vi "UHR-Fleezers Control (host) - Lorentz v3.vi"() -> ()   [LabVIEW 2014] (continued)
      n59 = call-poly "VISA Configure Serial Port"("VISA resource name"=refnum<visa-resource-name> "COM7", "baud rate (9600)"=u32 115200, "stop bits (10: 1 bit)"=w226) -> ("VISA resource name out"=w225:refnum<visa-resource-name>, "error out"=w224:errorcluster)  [unwired: 4 in, 7 out]
      n60 = call-poly "VISA Configure Serial Port"("VISA resource name"=refnum<visa-resource-name> "COM5", "baud rate (9600)"=u32 115200, "stop bits (10: 1 bit)"=w232) -> ("VISA resource name out"=w229:refnum<visa-resource-name>, "error out"=w228:errorcluster)  [unwired: 4 in, 7 out]
      n61 = call-poly "VISA Configure Serial Port"("VISA resource name"=refnum<visa-resource-name> "COM4", "baud rate (9600)"=u32 115200, "stop bits (10: 1 bit)"=w234) -> ("VISA resource name out"=w231:refnum<visa-resource-name>, "error out"=w230:errorcluster)  [unwired: 4 in, 7 out]
      n62 = call-poly "VISA Configure Serial Port"("VISA resource name"=refnum<visa-resource-name> "COM6", "baud rate (9600)"=u32 115200, "stop bits (10: 1 bit)"=w238) -> ("VISA resource name out"=w236:refnum<visa-resource-name>, "error out"=w237:errorcluster)  [unwired: 4 in, 7 out]
      n63 = call-poly "VISA Configure Serial Port"("VISA resource name"=refnum<visa-resource-name> "COM1") -> ("VISA resource name out"=w220:refnum<visa-resource-name>, "error out"=w240:errorcluster)  [unwired: 5 in, 8 out]
      "Stage Control Serial Error" <- w240
      n64 = local write "Blue Error Out"(w224) -> ()
    }
    frame Enabled {
    }
  }
  n65 = call "IMAQ Create"("Image Name"="APD 1 Image", "Image Type"=w35) -> ("New Image"=w52:T6)  [unwired: 3 in, 1 out]
  n66 = call "IMAQ Create"("Image Name"="APD 2 Image", "Image Type"=w35) -> ("New Image"=w51:T6)  [unwired: 3 in, 1 out]
  n67 = call "IMAQ Create"("Image Name"="APD 3 Image", "Image Type"=w35) -> ("New Image"=w34:T6)  [unwired: 3 in, 1 out]
  n68 = call "IMAQ Create"("Image Name"="Det. X Image", "Image Type"=w35) -> ("New Image"=w50:T6)  [unwired: 3 in, 1 out]
  n69 = call "IMAQ Create"("Image Name"="Det. Y Image", "Image Type"=w35) -> ("New Image"=w49:T6)  [unwired: 3 in, 1 out]
  n70 = Bundle("New Image"=w52, "New Image"=w51, "New Image"=w34, "New Image"=w50, "New Image"=w49) -> (w48:T35)  [unwired: 1 in]
  n71 = xnode "Open FPGA VI Reference"("resource name"=T28 "RIO0") -> ("FPGA VI Reference Out"=w29:T36, "error out"=w28:errorcluster)  [unwired: 1 in]
  n72 = xnode "Invoke Method"("FPGA VI Reference In"=w29, "error in"=w28) -> ("FPGA VI Reference Out"=w9:T36, "error out"=→"FPGA error out":errorcluster)
  n73 = Subtract(x=w7, y="Maximum Delta\n(MHz)") -> (x-y=w5:dbl)
  n74 = Bundle By Name(cluster=T24 {"Minimum"=60.0, "Maximum"=90.0, "Increment"=1.0} ("Min Max Inc"), "Minimum"=w5, "Maximum"=w7) -> (w4:T24)
  n75 = node-c288() -> (w55:T37)  [unwired: 4 in]
  n76 = timed-loop "Run Scripts, including: stage motion" {
    tunnel: w58 -> [w251]
    tunnel: w12 -> [w252]
    tunnel: [w252] -> w57
    tunnel: [w251] -> w56
    timing: w55 -> [_]
    timing-out: [_] -> w54
    tunnel: w46 -> [w250]
    tunnel: w47 -> [w249]
    tunnel: w42 -> [w246]
    tunnel: w41 -> [w245]
    tunnel: w40 -> [w247]
    tunnel: w39 -> [w248]
    tunnel: w31 -> [w244]
    tunnel: w24 -> [w243]
    tunnel: w11 -> [w242]
    tunnel: w10 -> [w241]
    stop <- w253 stop-if-true
    n77 = node-c288() -> ()  [unwired: 1 in, 1 out]
    n78 = event shown="[17] \"Got Bead 1\": Value Change" {
      selector: _ -> [_ _ _ _ _ _ _ _ _ _ _ _ _ _ _ _ _ _ _ _ _ _ _ _ _ _ _ _]
      dyn-events: _ -> [_ _ _ _ _ _ _ _ _ _ _ _ _ _ _ _ _ _ _ _ _ _ _ _ _ _ _ _]
      timeout: _ -> [_ _ _ _ _ _ _ _ _ _ _ _ _ _ _ _ _ _ _ _ _ _ _ _ _ _ _ _]
      tunnel: ["Set Position" "Move to Position" _ _ _ _ _ _ "Read Harvard" _ _ _ _ _ _ _ _ "Got Bead 1" "Force FB Data\nScript" _ "Got Bead 2" _ "Take Stepping Data" _ "Take Detection Laser\nImage" _ _ _] -> _
      tunnel: [_ _ _ _ _ _ _ _ _ _ _ _ _ _ _ _ _ _ _ _ _ _ _ _ _ _ w1180 _] -> w253
      tunnel: w251 -> [w272 w280 w293 w323 _ _ _ _ _ w460 w494 w520 w552 w641 w670 w802 w829 _ w871 _ _ _ _ _ _ _ _ _]
      tunnel: w252 -> [w273 w281 w294 w324 _ _ _ _ _ w461 w495 w521 w553 w642 w671 w803 w830 _ w872 _ _ _ _ _ _ _ _ _]
      tunnel: w250 -> [_ _ _ _ _ _ _ _ w445 _ _ _ _ _ _ _ _ _ _ _ _ _ _ _ _ _ _ _]
      tunnel: w249 -> [_ _ _ _ _ _ _ _ w444 _ _ _ _ _ _ _ _ _ _ _ _ _ _ _ _ _ _ _]
      tunnel: w248 -> [_ _ _ _ _ _ _ _ _ _ _ _ _ _ _ _ _ _ _ _ _ _ _ _ _ _ _ _]
      tunnel: w247 -> [_ _ _ _ _ _ _ _ _ _ _ _ _ _ _ _ _ _ _ _ _ _ _ _ _ _ _ _]
      tunnel: w246 -> [_ _ _ _ _ _ _ _ _ _ _ _ _ _ _ _ _ _ _ _ _ _ _ _ _ _ _ _]
      tunnel: w245 -> [_ _ _ _ _ _ _ _ _ _ _ _ _ _ _ _ _ _ _ _ _ _ _ _ _ _ _ _]
      tunnel: w244 -> [_ _ _ _ w351 w358 w386 w405 _ _ _ _ _ _ _ _ _ _ _ _ _ _ _ _ _ _ w1179 _]
      tunnel: w243 -> [_ _ _ _ _ _ _ _ _ _ _ _ _ _ _ _ _ _ _ _ _ _ _ _ _ w1046 _ _]
      tunnel: w242 -> [_ _ _ _ _ _ _ _ _ _ _ _ _ _ _ _ _ _ _ _ _ _ _ _ _ _ _ w1190]
      tunnel: w241 -> [_ _ _ _ _ _ _ _ _ _ _ _ _ _ _ _ _ _ _ _ _ _ _ _ _ _ _ w1185]
      tunnel: [_ _ _ _ _ _ _ _ _ _ _ _ _ _ _ _ _ _ _ _ _ "Get New Beads" _ _ _ _ _ _] -> _
      event "Set Position", "Set Position 2", "Set Position 3", "Set Position 4", "Set Position 5", "Set Position 1", "Set Position 6": Value Change {
        n79 = event-data() -> ()  [unwired: 1 in, 5 out]
        n80 = Build Array("Set Position 1", "Set Position 2", "Set Position 3", "Set Position 4", "Set Position 5", "Set Position 6") -> (w271:bool[])
        n81 = Boolean Array To Number(Boolean array=w271) -> (number=w270:u32)
        n82 = Logarithm Base 2(1:w270) -> (0:w262:dbl)
        n83 = call "Read Stage Position.vi"("error in"=w272, "VISA resource name in"=w273) -> ("Current Position"=w277:cluster{dbl, dbl, dbl}, "error out"=w276:errorcluster)  [unwired: 2 out]
        n84 = Decrement(x="Position") -> (x-1=w260:dbl)
        n85 = Greater Or Equal?(x=w262, y=0.0) -> (x >= y?=w263:bool)
        n86 = Cluster To Array(cluster=w277) -> (array=w274:dbl[])
        n87 = local write "Stage Control Serial Error"(w276) -> ()
        n88 = Select(t=w262, s=w263, f=w260) -> (s? t:f=w259:dbl)
        n89 = Increment(x=w259) -> (x+1=w258:dbl)
        n90 = Build Array (concatenate)(w258, w274) -> (w257:dbl[])
        n91 = Replace Array Subset(array="Saved Stage Positions", new element=w257, index (row)=w259) -> (w275:dbl[][])  [unwired: 1 in]
        n92 = local write "Saved Stage Positions"(w275) -> ()
      }
      event "Move to Position": Value Change {
        n93 = event-data() -> ()  [unwired: 1 in, 5 out]
        n94 = flat-sequence {
          tunnel: w281 -> [w285]
          tunnel: w280 -> [w284]
          frame #0 {
            n95 = local read "Saved Stage Positions"() -> (w287:dbl[][])
            n96 = local read "Position"() -> (w286:dbl)
            n97 = local write "Stage Moving"(TRUE ("Stage Moving")) -> ()
            n98 = call "move to saved stage position.vi"("error in"=w284, "Stage VISA resource name in"=w285, "Position"=w286, "Saved Stage Positions"=w287) -> ("error out"=w283:errorcluster)  [unwired: 1 out]
            n99 = local write "Stage Control Serial Error"(w283) -> ()
          }
          frame #1 {
            n100 = call <vilib>:"Beep.vi"() -> ()  [unwired: 3 in, 9 out]
            n101 = local write "Stage Moving"(FALSE ("Stage Moving")) -> ()
          }
        }
      }
      event "Move Cap. 1 (DNA Bottom)": Value Change {
        n102 = event-data() -> ()  [unwired: 1 in, 5 out]
        n103 = local write "Move Cap. 1 (DNA Bottom)"(FALSE ("Move Cap. 1 (DNA Right)")) -> ()
        n104 = flat-sequence {
          tunnel: w293 -> [w296]
          tunnel: w294 -> [w297]
          tunnel: [w297] -> w291
          tunnel: [w296] -> w290
          tunnel: w291 -> [w299]
          tunnel: w290 -> [w298]
          frame #0 {
            n105 = property on="Sample Channel\nFlow" class="Bool (strict)"("Val(Sgnl)"="Cap 1 Samp Flow ON") -> ()  [unwired: 2 in, 2 out]
          }
          frame #1 {
            n106 = local read "Saved Stage Positions"() -> (w309:dbl[][])
            n107 = local write "Stage Moving"(TRUE ("Stage Moving")) -> ()
            n108 = Array Subset(array=w309, index (row)=0 ("index"), length (row)=1 ("length"), index (col)=1 ("index"), length (col)=3 ("length")) -> (w306:dbl[][])
            n109 = Reshape Array(w306, 3 ("dimension size")) -> (w304:dbl[])
            n110 = Array To Cluster(array=w304) -> (cluster=w303:cluster{"[0]":dbl, "[1]":dbl, "[2]":dbl})
            n111 = call "Set Stage Position.vi"("Position"=w303, "error in"=w298, "VISA resource name in"=w299) -> ("error out"=w302:errorcluster)  [unwired: 2 out]
            n112 = local write "Stage Control Serial Error"(w302) -> ()
          }
          frame #2 {
            n113 = local write "Stage Moving"(FALSE ("Stage Moving")) -> ()
            n114 = case shown="True" "Cap 1 Flow ON" {
              frame False {
              }
              frame True {
                n115 = property on="Inject Pump 1" class="Bool (strict)"("Val(Sgnl)"=TRUE ("Value (Signaling)")) -> ()  [unwired: 2 in, 2 out]
              }
            }
            n116 = call <vilib>:"Beep.vi"() -> ()  [unwired: 3 in, 9 out]
          }
          frame #3 {
            n117 = property on="Sample Channel\nFlow" class="Bool (strict)"("Val(Sgnl)"=FALSE ("Value (Signaling)")) -> ()  [unwired: 2 in, 2 out]
            n118 = local read "Cap. 2 BD T1?\n(ADig T1, DNA T2)"() -> (w316:bool)
            n119 = case shown="True" w316 {
              tunnel: "Cap 1 T ON" -> [w318 w319]
              frame False {
                n120 = property on="Trap 1 (ON/OFF)" class="Bool (strict)"("Val(Sgnl)"=w318) -> ()  [unwired: 2 in, 2 out]
              }
              frame True {
                n121 = property on="Trap 2 (ON/OFF)" class="Bool (strict)"("Val(Sgnl)"=w319) -> ()  [unwired: 2 in, 2 out]
              }
            }
            n122 = property on="Got Bead 2" class="Bool"("Key Focus"=TRUE) -> ()  [unwired: 2 in, 2 out]
          }
        }
      }
      event "Move Cap. 2 (ADig Top)": Value Change {
        n123 = event-data() -> ()  [unwired: 1 in, 5 out]
        n124 = local write "Move Cap. 2 (ADig Top)"(FALSE ("Move Cap. 2 (ADig Left)")) -> ()
        n125 = flat-sequence {
          tunnel: w323 -> [w326]
          tunnel: w324 -> [w327]
          tunnel: [w327] -> w321
          tunnel: [w326] -> w320
          tunnel: w321 -> [w330]
          tunnel: w320 -> [w329]
          frame #0 {
            n126 = property on="Sample Channel\nFlow" class="Bool (strict)"("Val(Sgnl)"="Cap 2 Samp Flow ON") -> ()  [unwired: 2 in, 2 out]
          }
          frame #1 {
            w328 = FALSE ("Value (Signaling)")
            n127 = local read "Saved Stage Positions"() -> (w340:dbl[][])
            n128 = local write "Stage Moving"(TRUE ("Stage Moving")) -> ()
            n129 = Array Subset(array=w340, index (row)=1 ("index"), length (row)=1 ("length"), index (col)=1 ("index"), length (col)=3 ("length")) -> (w337:dbl[][])
            n130 = Reshape Array(w337, 3 ("dimension size")) -> (w335:dbl[])
            n131 = property on="Trap 1 (ON/OFF)" class="Bool (strict)"("Val(Sgnl)"=w328) -> ()  [unwired: 2 in, 2 out]
            n132 = property on="Trap 1 (ON/OFF)" class="Bool (strict)"("Val(Sgnl)"=w328) -> ()  [unwired: 2 in, 2 out]
            n133 = Array To Cluster(array=w335) -> (cluster=w334:cluster{"[0]":dbl, "[1]":dbl, "[2]":dbl})
            n134 = call "Set Stage Position.vi"("Position"=w334, "error in"=w329, "VISA resource name in"=w330) -> ("error out"=w333:errorcluster)  [unwired: 2 out]
            n135 = local write "Stage Control Serial Error"(w333) -> ()
          }
          frame #2 {
            n136 = local write "Stage Moving"(FALSE ("Stage Moving")) -> ()
            n137 = call <vilib>:"Beep.vi"() -> ()  [unwired: 3 in, 9 out]
            n138 = case shown="True" "Cap 2 Flow ON" {
              frame False {
              }
              frame True {
                n139 = property on="Inject Pump 3" class="Bool (strict)"("Val(Sgnl)"=TRUE ("Value (Signaling)")) -> ()  [unwired: 2 in, 2 out]
              }
            }
          }
          frame #3 {
            n140 = property on="Sample Channel\nFlow" class="Bool (strict)"("Val(Sgnl)"=FALSE ("Value (Signaling)")) -> ()  [unwired: 2 in, 2 out]
            n141 = case shown="False" "Cap. 2 BD T1?\n(ADig T1, DNA T2)" {
              tunnel: "Cap 2 T ON" -> [w349 w350]
              frame False {
                n142 = property on="Trap 2 (ON/OFF)" class="Bool (strict)"("Val(Sgnl)"=w349) -> ()  [unwired: 2 in, 2 out]
              }
              frame True {
                n143 = property on="Trap 1 (ON/OFF)" class="Bool (strict)"("Val(Sgnl)"=w350) -> ()  [unwired: 2 in, 2 out]
              }
            }
            n144 = property on="Got Bead 1" class="Bool"("Key Focus"=TRUE) -> ()  [unwired: 2 in, 2 out]
          }
        }
      }
      event "Send string\nto Blue Laser": Value Change {
        n145 = event-data() -> ()  [unwired: 1 in, 5 out]
        n146 = flat-sequence {
          tunnel: w351 -> [w352]
          frame #0 {
            n147 = call "serial write macro.vi"("String"="command string", "Delay (ms)"="Delay (ms)", "VISA resource name"=w352) -> ("read buffer"=→"read blue buffer":string, "error out"=→"Blue Error Out":errorcluster)  [unwired: 1 out]
            "command string sent" <- "command string"
          }
          frame #1 {
            n148 = local write "Send string\nto Blue Laser"(FALSE ("Send string")) -> ()
          }
        }
      }
      event "Get Blue Laser State": Value Change {
        n149 = event-data() -> ()  [unwired: 1 in, 5 out]
        n150 = local read "Delay (ms)"() -> (w359:i32)
        n151 = flat-sequence {
          tunnel: w359 -> [w367]
          tunnel: w358 -> [w370]
          tunnel: [w368] -> w363
          tunnel: [w367] -> w362
          tunnel: [w377] -> w361
          tunnel: [w374] -> w360
          tunnel: w363 -> [w375]
          tunnel: w362 -> [w374]
          tunnel: w361 -> [w383]
          tunnel: w360 -> [w381]
          frame #0 {
            w365 = "l?"
            n152 = local write "command string sent"(w365) -> ()
            n153 = call "serial write macro.vi"("String"=w365, "Delay (ms)"=w367, "VISA resource name"=w370) -> ("read buffer"=w366:string, "VISA resource name out"=w368:refnum<visa-resource-name>)  [unwired: 1 out]
            n154 = Decimal String To Number(string=w366) -> (number=w369:i32)  [unwired: 2 in, 1 out]
            n155 = Not Equal To 0?(x=w369) -> (x != 0?=→"Laser On":bool)
            n156 = local write "read blue buffer"(w366) -> ()
          }
          frame #1 {
            w372 = "games?" ("String")
            n157 = local write "command string sent"(w372) -> ()
            n158 = call "serial write macro.vi"("String"=w372, "Delay (ms)"=w374, "VISA resource name"=w375) -> ("read buffer"=w373:string, "VISA resource name out"=w377:refnum<visa-resource-name>)  [unwired: 1 out]
            n159 = Decimal String To Number(string=w373) -> (number=w376:i32)  [unwired: 2 in, 1 out]
            n160 = local write "read blue buffer"(w373) -> ()
            n161 = Not Equal To 0?(x=w376) -> (x != 0?=→"Analog Modulation":bool)
          }
          frame #2 {
            w379 = "gdmes?" ("String")
            n162 = local write "command string sent"(w379) -> ()
            n163 = call "serial write macro.vi"("String"=w379, "Delay (ms)"=w381, "VISA resource name"=w383) -> ("read buffer"=w380:string)  [unwired: 2 out]
            n164 = Decimal String To Number(string=w380) -> (number=w382:i32)  [unwired: 2 in, 1 out]
            n165 = Not Equal To 0?(x=w382) -> (x != 0?=→"Digital Modulation":bool)
            n166 = local write "read blue buffer"(w380) -> ()
          }
          frame #3 {
            n167 = local write "Get Blue Laser State"(FALSE) -> ()
          }
        }
      }
      event "Blue Laser Power (mW)\n(Constant Power Mode)", "Blue Laser Modulation\nPower (mW)": Value Change {
        n168 = event-data() -> ()  [unwired: 1 in, 5 out]
        n169 = flat-sequence {
          tunnel: w386 -> [w392]
          tunnel: [w390] -> w385
          tunnel: w385 -> [w399]
          frame #0 {
            n170 = local read "Delay (ms)"() -> (w391:i32)
            n171 = Concatenate Strings("slmp " ("string"), "Blue Laser Modulation\nPower (mW)") -> (w387:string)
            n172 = call "serial write macro.vi"("String"=w387, "Delay (ms)"=w391, "VISA resource name"=w392) -> ("read buffer"=w388:string, "error out"=w389:errorcluster, "VISA resource name out"=w390:refnum<visa-resource-name>)
            n173 = local write "command string sent"(w387) -> ()
            n174 = local write "read blue buffer"(w388) -> ()
            n175 = local write "Blue Error Out"(w389) -> ()
          }
          frame #1 {
            n176 = local read "Delay (ms)"() -> (w398:i32)
            n177 = Concatenate Strings("p " ("string"), "Blue Laser Power (mW)\n(Constant Power Mode)") -> (w395:string)
            n178 = call "serial write macro.vi"("String"=w395, "Delay (ms)"=w398, "VISA resource name"=w399) -> ("read buffer"=w396:string, "error out"=w397:errorcluster)  [unwired: 1 out]
            n179 = local write "command string sent"(w395) -> ()
            n180 = local write "read blue buffer"(w396) -> ()
            n181 = local write "Blue Error Out"(w397) -> ()
          }
        }
      }
      event "Laser interlacing mode", "Blue Laser Modulation Mode", "Blue Laser ON": Value Change {
        n182 = event-data() -> ()  [unwired: 1 in, 5 out]
        n183 = flat-sequence {
          tunnel: w405 -> [w410]
          tunnel: [w409] -> w402
          tunnel: [w415] -> w404
          tunnel: w402 -> [w418]
          tunnel: w404 -> [w430]
          tunnel: [w424] -> w403
          tunnel: w403 -> [w437]
          frame #0 {
            n184 = local read "Blue Laser ON"() -> (w407:bool)
            n185 = local read "Delay (ms)"() -> (w408:i32)
            n186 = case shown="False" w407 {
              tunnel: ["l0" "l1"] -> w406
              frame False {
              }
              frame True {
              }
            }
            n187 = call "serial write macro.vi"("String"=w406, "Delay (ms)"=w408, "VISA resource name"=w410) -> ("error out"=w411:errorcluster, "VISA resource name out"=w409:refnum<visa-resource-name>)  [unwired: 1 out]
            n188 = local write "Blue Error Out"(w411) -> ()
          }
          frame #1 {
            n189 = local read "Laser interlacing mode"() -> (w420:enum32{"Laser ON", "Laser OFF", "Interlace"})
            n190 = case shown="\"Laser ON\"" w420 {
              tunnel: ["cp" "em" "l0"] -> w414
              frame "Laser ON" {
              }
              frame "Interlace" {
              }
              frame "Laser OFF", Default {
              }
            }
            n191 = local read "Delay (ms)"() -> (w419:i32)
            n192 = call "serial write macro.vi"("String"=w414, "Delay (ms)"=w419, "VISA resource name"=w418) -> ("read buffer"=w416:string, "error out"=w417:errorcluster, "VISA resource name out"=w415:refnum<visa-resource-name>)
            n193 = local write "command string sent"(w414) -> ()
            n194 = local write "read blue buffer"(w416) -> ()
            n195 = local write "Blue Error Out"(w417) -> ()
          }
          frame #2 {
            n196 = case shown="\"Analog Modulation\"" "Blue Laser Modulation Mode" {
              tunnel: ["sdmes 0" "sdmes 1" "sdmes 1"] -> w425
              frame "Analog Modulation" {
              }
              frame "Digital + Analog Modulation" {
              }
              frame "Digital Modulation", Default {
              }
            }
            n197 = local read "Delay (ms)"() -> (w428:i32)
            n198 = call "serial write macro.vi"("String"=w425, "Delay (ms)"=w428, "VISA resource name"=w430) -> ("read buffer"=w426:string, "error out"=w427:errorcluster, "VISA resource name out"=w424:refnum<visa-resource-name>)
            n199 = local write "command string sent"(w425) -> ()
            n200 = local write "read blue buffer"(w426) -> ()
            n201 = local write "Blue Error Out"(w427) -> ()
          }
          frame #3 {
            n202 = local read "Blue Laser Modulation Mode"() -> (w439:string)
            n203 = case shown="\"Digital Modulation\", Default" w439 {
              tunnel: ["sames 1" "sames 1" "sames 0"] -> w435
              frame "Analog Modulation" {
              }
              frame "Digital + Analog Modulation" {
              }
              frame "Digital Modulation", Default {
              }
            }
            n204 = local read "Delay (ms)"() -> (w438:i32)
            n205 = local write "command string sent"(w435) -> ()
            n206 = call "serial write macro.vi"("String"=w435, "Delay (ms)"=w438, "VISA resource name"=w437) -> ("read buffer"=w436:string, "error out"=w434:errorcluster)  [unwired: 1 out]
            n207 = local write "read blue buffer"(w436) -> ()
            n208 = local write "Blue Error Out"(w434) -> ()
          }
        }
      }
      event "Read Harvard": Value Change {
        n209 = event-data() -> ()  [unwired: 1 in, 5 out]
        n210 = Concatenate Strings("write buffer", "\r") -> (w447:string)
        n211 = VISA Write(VISA resource name=w445, write buffer=w447, error in (no error)=w444) -> (VISA resource name out=w456:refnum<visa-resource-name>, error out=w455:errorcluster)  [unwired: 1 out]
        n212 = stacked-sequence {
          tunnel: [w459] -> w454
          tunnel: w456 -> [w459]
          tunnel: w455 -> [w458]
          tunnel: [w458] -> w449
          frame #0 {
            n213 = Wait (ms)(milliseconds to wait=50) -> ()  [unwired: 1 out]
          }
        }
        n214 = property class="Instr"(reference=w454, error in=w449) -> (reference out=w453:refnum<visa-resource-name>, error out=w451:errorcluster, "Serial Settings:Number of Bytes at Serial Port"=w452:u32)
        "Serial Settings:Number of Bytes at Serial Port" <- w452
        n215 = VISA Read(VISA resource name=w453, byte count=w452, error in (no error)=w451) -> (read buffer=w450:string)  [unwired: 3 out]
        "read buffer" <- w450
        n216 = Fract/Exp String To Number(string=w450) -> ()  [unwired: 5 out]
      }
      event "+z", "-z": Value Change {
        n217 = event-data() -> ()  [unwired: 1 in, 5 out]
        n218 = flat-sequence {
          tunnel: w460 -> [w482]
          tunnel: w461 -> [w462]
          frame #0 {
            n219 = call "Read Stage Position.vi"("error in"=w482, "VISA resource name in"=w462) -> ("Current Position"=w467:cluster{dbl, dbl, dbl}, "error out"=w480:errorcluster, "VISA resource name out"=w481:refnum<visa-resource-name>)  [unwired: 1 out]
            n220 = local read "Saved Stage Positions"() -> (w491:dbl[][])
            n221 = Divide(x="z nudge increment (um)", y=1000.0) -> (x/y=w479:dbl)
            n222 = Boolean To (0,1)(Boolean="+z") -> (0, 1=w471:i16)
            n223 = Boolean To (0,1)(Boolean="-z") -> (0, 1=w472:i16)
            n224 = Array Subset(array=w491, index (row)=1 ("index"), length (row)=1 ("length"), index (col)=1 ("index"), length (col)=3 ("length")) -> (w488:dbl[][])
            n225 = Multiply(x=w471, y=w479) -> (x*y=w475:dbl)
            n226 = Multiply(x=w472, y=w479) -> (x*y=w473:dbl)
            n227 = Unbundle(w467) -> (w465:dbl, w464:dbl, w468:dbl)
            n228 = Negate(x=w473) -> (-x=w474:dbl)
            n229 = Reshape Array(w488, 3 ("dimension size")) -> (w486:dbl[])
            n230 = Add(x=w475, y=w474) -> (x+y=w476:dbl)
            n231 = Array To Cluster(array=w486) -> ()  [unwired: 1 out]
            n232 = Add(x=w476, y=w468) -> (x+y=w466:dbl)
            n233 = Bundle(cluster=w467, w465, w464, w466) -> (w463:cluster{dbl, dbl, dbl})
            n234 = call "Set Stage Position.vi"("Position"=w463, "error in"=w480, "VISA resource name in"=w481) -> ("error out"=w485:errorcluster)  [unwired: 2 out]
            n235 = local write "Stage Moving"(TRUE ("Stage Moving")) -> ()
            n236 = local write "Stage Control Serial Error"(w485) -> ()
          }
          frame #1 {
            n237 = local write "Stage Moving"(FALSE ("Stage Moving")) -> ()
          }
        }
      }
      event "-y", "+y": Value Change {
        n238 = event-data() -> ()  [unwired: 1 in, 5 out]
        n239 = flat-sequence {
          tunnel: w494 -> [w518]
          tunnel: w495 -> [w501]
          frame #0 {
            n240 = call "Read Stage Position.vi"("error in"=w518, "VISA resource name in"=w501) -> ("Current Position"=w504:cluster{dbl, dbl, dbl}, "error out"=w516:errorcluster, "VISA resource name out"=w517:refnum<visa-resource-name>)  [unwired: 1 out]
            n241 = Divide(x="y nudge increment (um", y=1000.0) -> (x/y=w515:dbl)
            n242 = Boolean To (0,1)(Boolean="+y") -> (0, 1=w507:i16)
            n243 = Boolean To (0,1)(Boolean="-y") -> (0, 1=w508:i16)
            n244 = Multiply(x=w507, y=w515) -> (x*y=w511:dbl)
            n245 = Multiply(x=w508, y=w515) -> (x*y=w509:dbl)
            n246 = Unbundle(w504) -> (w503:dbl, w498:dbl, w500:dbl)
            n247 = Negate(x=w509) -> (-x=w510:dbl)
            n248 = Add(x=w511, y=w510) -> (x+y=w512:dbl)
            n249 = Add(x=w512, y=w498) -> (x+y=w499:dbl)
            n250 = Bundle(cluster=w504, w503, w499, w500) -> (w502:cluster{dbl, dbl, dbl})
            n251 = call "Set Stage Position.vi"("Position"=w502, "error in"=w516, "VISA resource name in"=w517) -> ("error out"=w497:errorcluster)  [unwired: 2 out]
            n252 = local write "Stage Control Serial Error"(w497) -> ()
            n253 = local write "Stage Moving"(TRUE ("Stage Moving")) -> ()
          }
          frame #1 {
            n254 = local write "Stage Moving"(FALSE ("Stage Moving")) -> ()
          }
        }
      }
      event "-x", "+x": Value Change {
        n255 = event-data() -> ()  [unwired: 1 in, 5 out]
        n256 = flat-sequence {
          tunnel: w520 -> [w544]
          tunnel: w521 -> [w528]
          frame #0 {
            n257 = call "Read Stage Position.vi"("error in"=w544, "VISA resource name in"=w528) -> ("Current Position"=w530:cluster{dbl, dbl, dbl}, "error out"=w542:errorcluster, "VISA resource name out"=w543:refnum<visa-resource-name>)  [unwired: 1 out]
            n258 = Divide(x="x nudge increment (um)", y=1000.0) -> (x/y=w541:dbl)
            n259 = Boolean To (0,1)(Boolean="+x") -> (0, 1=w533:i16)
            n260 = Boolean To (0,1)(Boolean="-x") -> (0, 1=w534:i16)
            n261 = Multiply(x=w533, y=w541) -> (x*y=w537:dbl)
            n262 = Multiply(x=w534, y=w541) -> (x*y=w535:dbl)
            n263 = Unbundle(w530) -> (w522:dbl, w524:dbl, w527:dbl)
            n264 = Negate(x=w535) -> (-x=w536:dbl)
            n265 = Add(x=w537, y=w536) -> (x+y=w538:dbl)
            n266 = Add(x=w538, y=w522) -> (x+y=w523:dbl)
            n267 = Bundle(cluster=w530, w523, w524, w527) -> (w529:cluster{dbl, dbl, dbl})
            n268 = call "Set Stage Position.vi"("Position"=w529, "error in"=w542, "VISA resource name in"=w543) -> ("error out"=w525:errorcluster)  [unwired: 2 out]
            n269 = local write "Stage Control Serial Error"(w525) -> ()
            n270 = local write "Stage Moving"(TRUE ("Stage Moving")) -> ()
          }
          frame #1 {
            n271 = local write "Stage Moving"(FALSE ("Stage Moving")) -> ()
          }
        }
      }
      event "Cal/Data Acq. Spot": Value Change {
        # "Disabled by Ronen - we have our own way of controlling the location of calibration."
        n272 = event-data() -> ()  [unwired: 1 in, 5 out]
        n273 = flat-sequence {
          tunnel: w552 -> [w556]
          tunnel: w553 -> [w557]
          tunnel: [w557] -> w549
          tunnel: [w556] -> w548
          tunnel: w549 -> [w560]
          tunnel: w548 -> [w559]
          tunnel: ["Cal @ (MHz)"] -> w546
          tunnel: [w568] -> w550
          tunnel: w546 -> [w568]
          tunnel: w550 -> [w580]
          tunnel: ["W/ Offset 1"] -> w547
          tunnel: w550 -> [w601]
          tunnel: w547 -> [w599]
          frame #0 {
            n274 = property on="Sample Channel\nFlow" class="Bool (strict)"("Val(Sgnl)"="Daq spot flow on") -> ()  [unwired: 2 in, 2 out]
            n275 = Wait (ms)(milliseconds to wait=u32 250) -> ()  [unwired: 1 out]
          }
          frame #1 {
            n276 = disable-structure shown="Disabled" {
              disable-tunnel: w560 -> [w565 _]
              disable-tunnel: w559 -> [w564 _]
              frame Disabled {
                n277 = local read "Saved Stage Positions"() -> (w562:dbl[][])
                n278 = call "move to saved stage position.vi"("error in"=w564, "Stage VISA resource name in"=w565, "Position"="Cal Stage Position", "Saved Stage Positions"=w562) -> ("error out"=w563:errorcluster)  [unwired: 1 out]
                n279 = local write "Stage Control Serial Error"(w563) -> ()
              }
              frame Enabled {
              }
            }
            n280 = property on="Trap Delta (MHz)" class="DigNum (strict)"("Val(Sgnl)"="Cal @ (MHz)") -> ()  [unwired: 2 in, 2 out]
            n281 = local write "Stage Moving"(TRUE ("Stage Moving")) -> ()
          }
          frame #2 {
            n282 = local write "Stage Moving"(FALSE ("Stage Moving")) -> ()
            n283 = property on="Sample Channel\nFlow" class="Bool (strict)"("Val(Sgnl)"="Flow ON during cal?") -> ()  [unwired: 2 in, 2 out]
            n284 = call <vilib>:"Beep.vi"() -> ()  [unwired: 3 in, 9 out]
          }
          frame #3 {
            n285 = Wait (ms)(milliseconds to wait=u32 1000) -> ()  [unwired: 1 out]
          }
          frame #4 {
            n286 = case shown="True" "Active cal after cal?" {
              frame False {
              }
              frame True {
                n287 = local write "Active Cal"(TRUE ("Active Cal")) -> ()
                n288 = Wait (ms)(milliseconds to wait=u32 8000) -> ()  [unwired: 1 out]
              }
            }
          }
          frame #5 {
            n289 = property on="Save Calibration" class="Bool (strict)"("Val(Sgnl)"=TRUE ("Value (Signaling)")) -> ()  [unwired: 2 in, 2 out]
          }
          frame #6 {
            n290 = Wait (ms)(milliseconds to wait=u32 2000) -> ()  [unwired: 1 out]
          }
          frame #7 {
            # "Check to see if \nsaving done"
            n291 = while {
              stop <- w576 stop-if-true
              n292 = local read "Saving..."() -> (w577:bool)
              n293 = Wait (ms)(milliseconds to wait=u32 100) -> ()  [unwired: 1 out]
              n294 = Not(x=w577) -> (.not. x?=w576:bool)
            }
          }
          frame #8 {
            n295 = case shown="True" "W/ Offset 1" {
              tunnel: w580 -> [_ w581]
              frame False {
              }
              frame True {
                n296 = stacked-sequence {
                  tunnel: w581 -> [_ _ _ _ _ _ _ w598]
                  frame #0 {
                    n297 = property on="Trap Delta (MHz)" class="DigNum (strict)"("Val(Sgnl)"="Offset 1 Start (MHz)") -> ()  [unwired: 2 in, 2 out]
                    n298 = Replace Array Subset(array=u32[] [0] ("Index Values"), new element="Offset 1 Set", index=0) -> (w583:u32[])
                    n299 = property on="Saved AOD Raster Scan Parameter Sets" class="Arr (strict)"("Index Values"=w583) -> ()  [unwired: 2 in, 2 out]
                    n300 = property on="manual raster set" class="Ring (strict)"("Value"="Offset 1 Set") -> ()  [unwired: 2 in, 2 out]
                  }
                  frame #1 {
                    n301 = Wait (ms)(milliseconds to wait=u32 200) -> ()  [unwired: 1 out]
                  }
                  frame #2 {
                    n302 = property on="Load parameters" class="Bool (strict)"("Val(Sgnl)"=TRUE ("Value (Signaling)")) -> ()  [unwired: 2 in, 2 out]
                  }
                  frame #3 {
                    n303 = Wait (ms)(milliseconds to wait=u32 200) -> ()  [unwired: 1 out]
                  }
                  frame #4 {
                    n304 = property on="Trap Raster Scan" class="Bool (strict)"("Val(Sgnl)"=TRUE ("Value (Signaling)")) -> ()  [unwired: 2 in, 2 out]
                  }
                  frame #5 {
                    n305 = Wait (ms)(milliseconds to wait=u32 2000) -> ()  [unwired: 1 out]
                  }
                  frame #6 {
                    n306 = while {
                      stop <- w595 stop-if-true
                      n307 = local read "Raster Scanning..."() -> (w597:bool)
                      n308 = local read "Saving..."() -> (w593:bool)
                      n309 = Wait (ms)(milliseconds to wait=u32 100) -> ()  [unwired: 1 out]
                      n310 = Not(x=w593) -> (.not. x?=w592:bool)
                      n311 = Not(x=w597) -> (.not. x?=w594:bool)
                      n312 = And(x=w594, y=w592) -> (x .and. y?=w595:bool)
                    }
                  }
                  frame #7 {
                    n313 = property on="Trap Delta (MHz)" class="DigNum (strict)"("Val(Sgnl)"=w598) -> ()  [unwired: 2 in, 2 out]
                  }
                }
              }
            }
          }
          frame #9 {
            n314 = local read "Save ave N"() -> (w600:dbl)
            n315 = case shown="True" "W/ Offset 2" {
              tunnel: w601 -> [_ w608]
              tunnel: w600 -> [_ w607]
              tunnel: w599 -> [w603 _]
              frame False {
                n316 = case shown="False" w603 {
                  frame False {
                    n317 = Multiply(x="Cal read wait (s)", y=u32 1000 ("milliseconds to wait")) -> (x*y=w605:u32)
                    n318 = Wait (ms)(milliseconds to wait=w605) -> ()  [unwired: 1 out]
                  }
                  frame True {
                  }
                }
              }
              frame True {
                n319 = stacked-sequence {
                  tunnel: w608 -> [_ _ _ _ _ _ _ _ _ w629 _ _]
                  tunnel: w607 -> [_ _ _ _ _ _ _ _ _ w627 _ _]
                  frame #0 {
                    n320 = property on="Save ave N" class="DigNum (strict)"("Val(Sgnl)"=1.0 ("Value (Signaling)")) -> ()  [unwired: 2 in, 2 out]
                  }
                  frame #1 {
                    n321 = Wait (ms)(milliseconds to wait=u32 500) -> ()  [unwired: 1 out]
                  }
                  frame #2 {
                    n322 = property on="Trap Delta (MHz)" class="DigNum (strict)"("Val(Sgnl)"="Offset 2 Start (MHz)") -> ()  [unwired: 2 in, 2 out]
                    n323 = Replace Array Subset(array=u32[] [0] ("Index Values"), new element="Offset 2 Set", index=0) -> (w613:u32[])
                    n324 = property on="Saved AOD Raster Scan Parameter Sets" class="Arr (strict)"("Index Values"=w613) -> ()  [unwired: 2 in, 2 out]
                  }
                  frame #3 {
                    n325 = Wait (ms)(milliseconds to wait=u32 500) -> ()  [unwired: 1 out]
                  }
                  frame #4 {
                    n326 = property on="Load parameters" class="Bool (strict)"("Val(Sgnl)"=TRUE ("Value (Signaling)")) -> ()  [unwired: 2 in, 2 out]
                  }
                  frame #5 {
                    n327 = Wait (ms)(milliseconds to wait=u32 500) -> ()  [unwired: 1 out]
                  }
                  frame #6 {
                    n328 = property on="Trap Raster Scan" class="Bool (strict)"("Val(Sgnl)"=TRUE ("Value (Signaling)")) -> ()  [unwired: 2 in, 2 out]
                  }
                  frame #7 {
                    n329 = Wait (ms)(milliseconds to wait=u32 2000) -> ()  [unwired: 1 out]
                  }
                  frame #8 {
                    n330 = while {
                      stop <- w622 stop-if-true
                      n331 = local read "Raster Scanning..."() -> (w625:bool)
                      n332 = local read "Saving..."() -> (w623:bool)
                      n333 = Wait (ms)(milliseconds to wait=u32 100) -> ()  [unwired: 1 out]
                      n334 = Not(x=w623) -> (.not. x?=w621:bool)
                      n335 = Not(x=w625) -> (.not. x?=w624:bool)
                      n336 = And(x=w624, y=w621) -> (x .and. y?=w622:bool)
                    }
                  }
                  frame #9 {
                    n337 = property on="Trap Delta (MHz)" class="DigNum (strict)"("Val(Sgnl)"=w629) -> ()  [unwired: 2 in, 2 out]
                    n338 = property on="Saved AOD Raster Scan Parameter Sets" class="Arr (strict)"("Index Values"=u32[] [0]) -> ()  [unwired: 2 in, 2 out]
                    n339 = property on="Save ave N" class="DigNum (strict)"("Val(Sgnl)"=w627) -> ()  [unwired: 2 in, 2 out]
                  }
                  frame #10 {
                    n340 = Wait (ms)(milliseconds to wait=u32 500) -> ()  [unwired: 1 out]
                  }
                  frame #11 {
                    n341 = property on="Load parameters" class="Bool (strict)"("Val(Sgnl)"=TRUE ("Value (Signaling)")) -> ()  [unwired: 2 in, 2 out]
                  }
                }
              }
            }
          }
          frame #10 {
            # "Added by Ronen for flow calibration"
            n342 = case shown="True" "Flow based calibration?" {
              frame False {
              }
              frame True {
                n343 = stacked-sequence {
                  frame #0 {
                    n344 = local write "Flow Cal"(TRUE) -> ()
                  }
                  frame #1 {
                  }
                  frame #2 {
                    n345 = Wait (ms)(milliseconds to wait=u32 8000) -> ()  [unwired: 1 out]
                  }
                }
              }
            }
          }
          frame #11 {
            n346 = property on="Read Cal" class="Bool (strict)"("Val(Sgnl)"=TRUE ("Value (Signaling)")) -> ()  [unwired: 2 in, 2 out]
          }
          frame #12 {
            n347 = Wait (ms)(milliseconds to wait=u32 1000) -> ()  [unwired: 1 out]
          }
          frame #13 {
            n348 = property on="Fish for Tether" class="Bool (strict)"("Val(Sgnl)"="Fish after cal?") -> ()  [unwired: 2 in, 2 out]
          }
        }
        n349 = local write "Cal/Data Acq. Spot"(FALSE ("Cal/Data Acq. Spot")) -> ()
      }
      event "Dump Beads": Value Change {
        n350 = event-data() -> ()  [unwired: 1 in, 5 out]
        n351 = flat-sequence {
          tunnel: ["Dump spot flow on?"] -> w638
          tunnel: [w649] -> w639
          tunnel: w638 -> [w649]
          tunnel: w642 -> [w654]
          tunnel: w641 -> [w653]
          tunnel: [w651] -> w640
          tunnel: w639 -> [w651]
          tunnel: w640 -> [w664]
          frame #0 {
            w643 = FALSE ("Value (Signaling)")
            n352 = local read "Saving..."() -> (w645:bool)
            n353 = local write "Dump Beads"(FALSE ("Dump Beads")) -> ()
            n354 = property on="Inject Pump 3" class="Bool (strict)"("Val(Sgnl)"=w643) -> ()  [unwired: 2 in, 2 out]
            n355 = property on="Inject Pump 1" class="Bool (strict)"("Val(Sgnl)"=w643) -> ()  [unwired: 2 in, 2 out]
            n356 = local write "Stop Saving"(w645) -> ()
          }
          frame #1 {
            w646 = FALSE ("Fl. Triggered...")
            n357 = case shown="True" "Dump spot flow on?" {
              frame False {
              }
              frame True {
                n358 = property on="Sample Channel\nFlow" class="Bool (strict)"("Val(Sgnl)"=TRUE ("Stage Moving")) -> ()  [unwired: 2 in, 2 out]
              }
            }
            n359 = local write "Fl. Triggered..."(w646) -> ()
            n360 = local write "Tether"(w646) -> ()
            n361 = property on="Green Laser ON" class="Bool (strict)"("Val(Sgnl)"=w646) -> ()  [unwired: 2 in, 2 out]
            n362 = property on="Trap Pos. FB ON" class="Bool (strict)"("Val(Sgnl)"=w646) -> ()  [unwired: 2 in, 2 out]
            n363 = property on="Trap Trig. Fl." class="Bool (strict)"("Val(Sgnl)"=w646) -> ()  [unwired: 2 in, 2 out]
            n364 = property on="Fl. Triggered..." class="Bool (strict)"("Val(Sgnl)"=w646) -> ()  [unwired: 2 in, 2 out]
            n365 = property on="Dip for Protein" class="Bool (strict)"("Val(Sgnl)"=w646) -> ()  [unwired: 2 in, 2 out]
            n366 = property on="Pause dwell" class="Bool (strict)"("Val(Sgnl)"=w646) -> ()  [unwired: 2 in, 2 out]
          }
          frame #2 {
            n367 = property on="Trap Pos. FB Offset Factor" class="DigNum (strict)"("Val(Sgnl)"=i64 0 ("Value (Signaling)")) -> ()  [unwired: 2 in, 2 out]
          }
          frame #3 {
            n368 = local read "Saved Stage Positions"() -> (w655:dbl[][])
            n369 = local write "Stage Moving"(TRUE ("Stage Moving")) -> ()
            n370 = Array Subset(array=w655, index (row)=3 ("index"), length (row)=1 ("length"), index (col)=1 ("index"), length (col)=3 ("length")) -> (w660:dbl[][])
            n371 = Reshape Array(w660, 3 ("dimension size")) -> (w658:dbl[])
            n372 = Array To Cluster(array=w658) -> (cluster=w657:cluster{"[0]":dbl, "[1]":dbl, "[2]":dbl})
            n373 = call "Set Stage Position.vi"("Position"=w657, "error in"=w653, "VISA resource name in"=w654) -> ()  [unwired: 3 out]
          }
          frame #4 {
            w665 = FALSE ("Value (Signaling)")
            n374 = case shown="True" w664 {
              frame False {
              }
              frame True {
                n375 = property on="Sample Channel\nFlow" class="Bool (strict)"("Val(Sgnl)"=FALSE ("Stage Moving")) -> ()  [unwired: 2 in, 2 out]
              }
            }
            n376 = property on="Trap 1 (ON/OFF)" class="Bool (strict)"("Val(Sgnl)"=w665) -> ()  [unwired: 2 in, 2 out]
            n377 = property on="Trap 2 (ON/OFF)" class="Bool (strict)"("Val(Sgnl)"=w665) -> ()  [unwired: 2 in, 2 out]
            n378 = call <vilib>:"Beep.vi"() -> ()  [unwired: 3 in, 9 out]
          }
          frame #5 {
            n379 = property on="Move Cap. 2 (ADig Top)" class="Bool (strict)"("Val(Sgnl)"=TRUE ("Value (Signaling)")) -> ()  [unwired: 2 in, 2 out]
            n380 = property on="Tab Control" class="TabCtl (strict)"("Val(Sgnl)"=T40."Status" ("Value (Signaling)")) -> ()  [unwired: 2 in, 2 out]
          }
        }
      }
      event "Dip for Protein": Value Change {
        n381 = event-data() -> ()  [unwired: 1 in, 5 out]
        n382 = case shown="True" "Dip for Protein" {
          tunnel: w671 -> [_ w673]
          tunnel: w670 -> [_ w672]
          frame False {
          }
          frame True {
            n383 = while {
              tunnel: w673 -> [w684]
              tunnel: w672 -> [w683]
              i -> [w678]
              stop <- w680 stop-if-true
              n384 = Increment(x=w678) -> (x+1=→"Dip #":i32)
              n385 = flat-sequence {
                tunnel: w683 -> [w695]
                tunnel: w684 -> [w696]
                tunnel: [w696] -> w688
                tunnel: [w695] -> w687
                tunnel: [w689] -> w674
                tunnel: [w701] -> w682
                tunnel: [w702] -> w681
                tunnel: w688 -> [w703]
                tunnel: w687 -> [w704]
                tunnel: [w699] -> w675
                tunnel: w674 -> [w699]
                tunnel: [w712] -> w686
                tunnel: w682 -> [w712]
                tunnel: [w711] -> w685
                tunnel: w681 -> [w711]
                tunnel: [w708] -> w679
                tunnel: [w707] -> w676
                tunnel: w675 -> [w707]
                tunnel: w685 -> [w732]
                tunnel: w686 -> [w733]
                tunnel: w679 -> [w734]
                tunnel: w676 -> [w731]
                tunnel: [w790] -> w680
                frame #0 {
                  n386 = local read "Trap Pos. FB ON"() -> (w689:bool)
                  n387 = Compound Arithmetic op=AND("Flow ON\nduring dip?", "FB OFF when \nflow ON", w689) -> (w690:bool)
                  n388 = case shown="True" "Move trap \nbefore dip move?" {
                    frame False {
                    }
                    frame True {
                      n389 = property on="Trap Delta (MHz)" class="DigNum (strict)"("Val(Sgnl)"="Dipping Delta (MHz)") -> ()  [unwired: 2 in, 2 out]
                    }
                  }
                  n390 = property on="Green Laser ON" class="Bool (strict)"("Val(Sgnl)"="Green ON\nbefore dip?") -> ()  [unwired: 2 in, 2 out]
                  n391 = property on="Sample Channel\nFlow" class="Bool (strict)"("Val(Sgnl)"="Flow ON\nduring dip?") -> ()  [unwired: 2 in, 2 out]
                  n392 = case shown="True" w690 {
                    frame False {
                    }
                    frame True {
                      n393 = property on="Trap Pos. FB ON" class="Bool (strict)"("Val(Sgnl)"=FALSE ("Value (Signaling)")) -> ()  [unwired: 2 in, 2 out]
                    }
                  }
                }
                frame #1 {
                  n394 = local read "Saved Stage Positions"() -> (w706:dbl[][])
                  n395 = local write "Cancel dwell"(FALSE ("Cancel dwell")) -> ()
                  n396 = call "move to saved stage position.vi"("error in"=w704, "Stage VISA resource name in"=w703, "Position"="Dip Stage \nPosition", "Saved Stage Positions"=w706) -> ("VISA resource name out"=w701:refnum<visa-resource-name>, "error out"=w702:errorcluster)
                }
                frame #2 {
                  n397 = node-c288() -> (w710:T37)  [unwired: 4 in]
                  n398 = timed-loop {
                    timing: w710 -> [_]
                    timing-out: [_] -> w709
                    tunnel: [w716] -> w708
                    i -> [w713]
                    stop <- w717 stop-if-true
                    n399 = node-c288() -> ()  [unwired: 1 in, 1 out]
                    n400 = Greater Or Equal?(x=w713, y="Dip Duration (s)") -> (x >= y?=w725:bool)
                    n401 = local read "Dip for Protein"() -> (w718:bool)
                    n402 = local read "Dump Beads"() -> (w715:bool)
                    n403 = local read "Cancel dwell"() -> (w724:bool)
                    n404 = local read "Pause dwell"() -> (w721:bool)
                    n405 = Not(x=w718) -> (.not. x?=w723:bool)
                    n406 = Compound Arithmetic op=OR(w724, w725, w723) -> (w722:bool)
                    n407 = Select(t=FALSE, s=w721, f=w722) -> (s? t:f=w719:bool)
                    n408 = Not(x=w715) -> (.not. x?=w714:bool)
                    n409 = node-c288() -> ()  [unwired: 1 in, 1 out]
                    n410 = And(x=w718, y=w714) -> (x .and. y?=w716:bool)
                    n411 = Or(x=w719, y=w715) -> (x .or. y?=w717:bool)
                    "Dip Time (s)" <- w713
                  }
                  n412 = node-c288(w709) -> ()  [unwired: 1 out]
                }
                frame #3 {
                  n413 = case shown="True" w734 {
                    tunnel: w733 -> [_ w739]
                    tunnel: w732 -> [_ w738]
                    tunnel: w731 -> [_ w735]
                    frame False {
                    }
                    frame True {
                      n414 = flat-sequence {
                        tunnel: w738 -> [w743]
                        tunnel: w739 -> [w744]
                        tunnel: [w744] -> w737
                        tunnel: [w743] -> w736
                        tunnel: w735 -> [w740]
                        tunnel: w737 -> [w754]
                        tunnel: w736 -> [w753]
                        tunnel: w735 -> [w762]
                        frame #0 {
                          n415 = local read "Sample Channel\nFlow"() -> (w742:bool)
                          n416 = case shown="True" w742 {
                            tunnel: "Flow ON \nduring return\nfrom dip?" -> [w745 w748]
                            tunnel: w740 -> [_ w747]
                            frame False {
                              n417 = case shown="True" w745 {
                                frame False {
                                }
                                frame True {
                                n418 = property on="Sample Channel\nFlow" class="Bool (strict)"("Val(Sgnl)"=TRUE ("Value (Signaling)")) -> ()  [unwired: 2 in, 2 out]
                                }
                              }
                            }
                            frame True {
                              n419 = case shown="False" w748 {
                                tunnel: w747 -> [w749 _]
                                frame False {
                                n420 = property on="Trap Pos. FB ON" class="Bool (strict)"("Val(Sgnl)"=w749) -> ()  [unwired: 2 in, 2 out]
                                n421 = property on="Sample Channel\nFlow" class="Bool (strict)"("Val(Sgnl)"=FALSE ("Value (Signaling)")) -> ()  [unwired: 2 in, 2 out]
                                }
                                frame True {
                                }
                              }
                            }
                          }
                        }
                        frame #1 {
                          # "For turning on green laser before stage reaches lower spot"
                          n422 = case shown="True" "Green ON\nafter start\nreturn?" {
                            frame False {
                            }
                            frame True {
                              n423 = flat-sequence {
                                frame #0 {
                                n424 = Multiply(x="Green delay after \nstart return (s)", y=1000.0) -> (x*y=w759:dbl)
                                n425 = Wait (ms)(milliseconds to wait=w759) -> ()  [unwired: 1 out]
                                }
                                frame #1 {
                                n426 = property on="Green Laser ON" class="Bool (strict)"("Val(Sgnl)"=TRUE ("Value (Signaling)")) -> ()  [unwired: 2 in, 2 out]
                                }
                              }
                            }
                          }
                          n427 = local read "Saved Stage Positions"() -> (w757:dbl[][])
                          n428 = local write "Cancel dwell"(FALSE ("Cancel dwell")) -> ()
                          n429 = call "move to saved stage position.vi"("error in"=w753, "Stage VISA resource name in"=w754, "Position"="Return Stage \nPosition", "Saved Stage Positions"=w757) -> ("error out"=w755:errorcluster)  [unwired: 1 out]
                          n430 = local write "Stage Control Serial Error"(w755) -> ()
                        }
                        frame #2 {
                          n431 = property on="Trap Pos. FB ON" class="Bool (strict)"("Val(Sgnl)"=w762) -> ()  [unwired: 2 in, 2 out]
                          n432 = case shown="True" "Green ON \nafter return?" {
                            frame False {
                            }
                            frame True {
                              n433 = property on="Green Laser ON" class="Bool (strict)"("Val(Sgnl)"=TRUE ("Value (Signaling)")) -> ()  [unwired: 2 in, 2 out]
                            }
                          }
                          n434 = case shown="True" "Move trap after return?" {
                            frame False {
                            }
                            frame True {
                              n435 = property on="Trap Delta (MHz)" class="DigNum (strict)"("Val(Sgnl)"="Dip Trap Delta 2 (MHz)") -> ()  [unwired: 2 in, 2 out]
                            }
                          }
                          n436 = case shown="True" "Save data after return?" {
                            frame False {
                            }
                            frame True {
                              n437 = property on="Start Saving" class="Bool (strict)"("Val(Sgnl)"=TRUE ("Value (Signaling)")) -> ()  [unwired: 2 in, 2 out]
                            }
                          }
                          n438 = property on="Sample Channel\nFlow" class="Bool (strict)"("Val(Sgnl)"="Flow ON\nduring daq?") -> ()  [unwired: 2 in, 2 out]
                        }
                        frame #3 {
                          n439 = node-c288() -> (w771:T37)  [unwired: 4 in]
                          n440 = timed-loop {
                            timing: w771 -> [_]
                            timing-out: [_] -> w770
                            i -> [w772]
                            stop <- w774 stop-if-true
                            n441 = node-c288() -> ()  [unwired: 1 in, 1 out]
                            n442 = local read "Dump Beads"() -> (w773:bool)
                            n443 = Greater Or Equal?(x=w772, y="Dwell Duration (s)") -> (x >= y?=w779:bool)
                            n444 = local read "Dip for Protein"() -> (w776:bool)
